vi "Actor Core.vi"(8 "error in":errorcluster, 11 "Actor in":refnum<class "EventLogger_Actor.lvclass">) -> (0 "error out":errorcluster, 3 "Actor out":refnum<class "Actor.lvclass">)   [LabVIEW 2014, in "EventLogger_Actor.lvlib" / "EventLogger_Actor.lvclass"]
uses:
  EventLogger_Actor.lvclass
  <vilib>/ActorFramework/Actor/Actor.lvclass
  EventLogger_Actor.lvclass/EventLogger_Actor.ctl
  <vilib>/ActorFramework/Actor/Actor.lvclass/Actor.ctl
  <vilib>/ActorFramework/Message Enqueuer/Message Enqueuer.lvclass/Message Enqueuer.ctl
  <vilib>/ActorFramework/Message Enqueuer/Init from Existing Queue.vi
  <vilib>/ActorFramework/Message Enqueuer/Enqueue.vi
  <vilib>/ActorFramework/Message Priority Queue/Priority Enqueue.vi
  <vilib>/ActorFramework/Message Enqueuer/Message Enqueuer.lvclass
  <vilib>/ActorFramework/Stop Msg/Stop Msg.lvclass
  EventLogger_Actor Messages/OpenLogs_Msg/OpenLogs_Msg.lvclass
panel:
  in  "ShowOnlyErrors":bool
  in  "Multicolumn Listbox":i32(listbox)
  out "StopLoop(Hidden)":bool
  in  "Stop":bool
  # "BSD 2-Clause License\n\nCopyright (c) 2018, Ajay www.digiajay.com\nAll rights reserved.\n\nRedistribution and use in source and binary forms, with or without\nmodification, are permitted provided that the following conditions are met:\n\n* Redistributions of source code must retain the above copyright notice, this\n  list of conditions and the following disclaimer.\n\n* Redistributions in binary form must reproduce the above copyright notice,\n  this list of conditions and the following disclaimer in the documentation\n  and/or other materials provided with the distribution.\n\nTHIS SOFTWARE IS PROVIDED BY THE COPYRIGHT HOLDERS AND CONTRIBUTORS \"AS IS\"\nAND ANY EXPRESS OR IMPLIED WARRANTIES, INCLUDING, BUT NOT LIMITED TO, THE\nIMPLIED WARRANTIES OF MERCHANTABILITY AND FITNESS FOR A PARTICULAR PURPOSE ARE\nDISCLAIMED. IN NO EVENT SHALL THE COPYRIGHT HOLDER OR CONTRIBUTORS BE LIABLE\nFOR ANY DIRECT, INDIRECT, INCIDENTAL, SPECIAL, EXEMPLARY, OR CONSEQUENTIAL\nDAMAGES (INCLUDING, BUT NOT LIMITED TO, PROCUREMENT OF SUBSTITUTE GOODS OR\nSERVICES; LOSS OF USE, DATA, OR PROFITS; OR BUSINESS INTERRUPTION) HOWEVER\nCAUSED AND ON ANY THEORY OF LIABILITY, WHETHER IN CONTRACT, STRICT LIABILITY,\nOR TORT (INCLUDING NEGLIGENCE OR OTHERWISE) ARISING IN ANY WAY OUT OF THE USE\nOF THIS SOFTWARE, EVEN IF ADVISED OF THE POSSIBILITY OF SUCH DAMAGE."
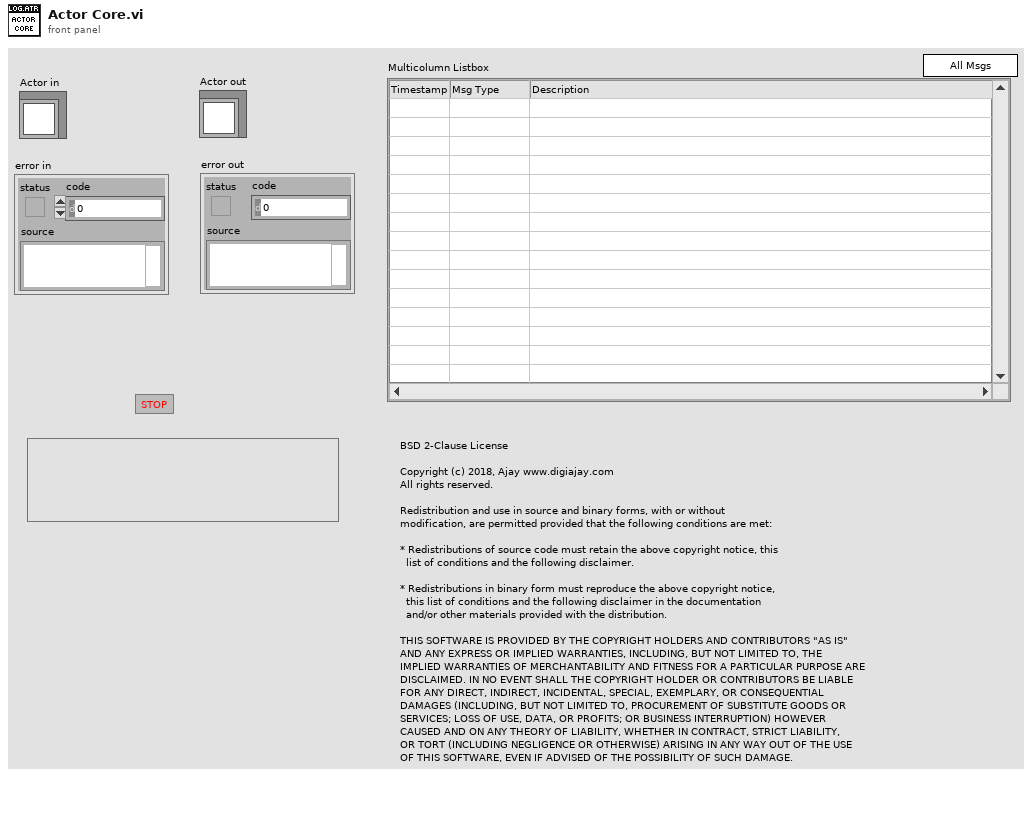
[diagram p1: front panel]
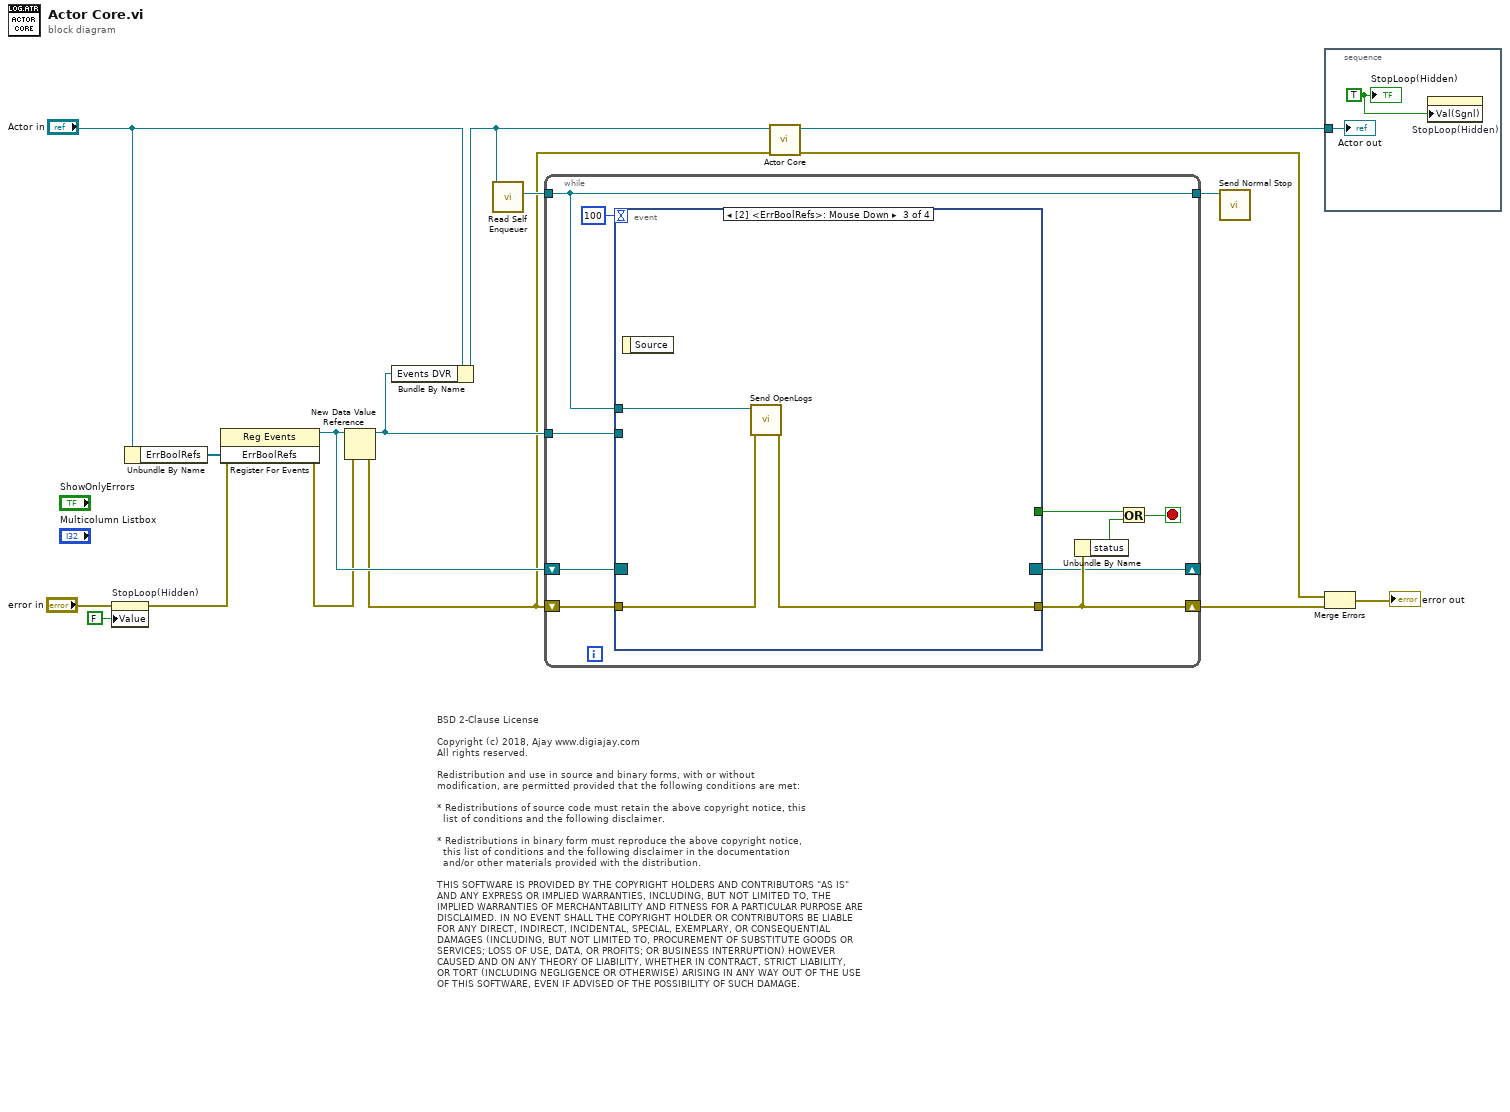
[diagram p0: block diagram]
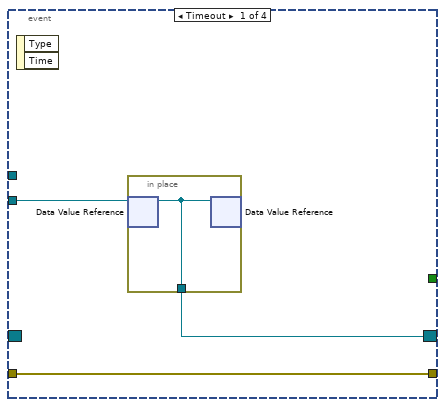
[diagram p2: hidden frame]
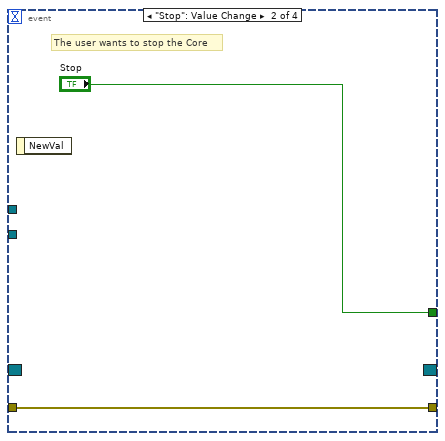
[diagram p3: hidden frame]
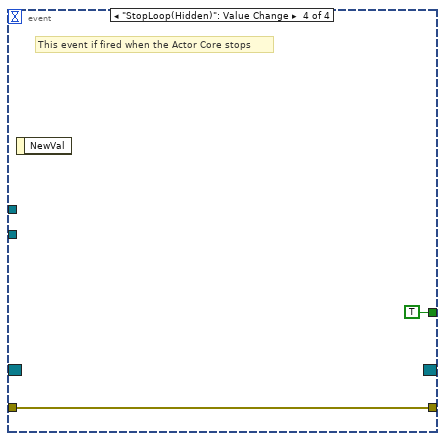
[diagram p4: hidden frame]
diagram:
  # "BSD 2-Clause License\n\nCopyright (c) 2018, Ajay www.digiajay.com\nAll rights reserved.\n\nRedistribution and use in source and binary forms, with or without\nmodification, are permitted provided that the following conditions are met:\n\n* Redistributions of source code must retain the above copyright notice, this\n  list of conditions and the following disclaimer.\n\n* Redistributions in binary form must reproduce the above copyright notice,\n  this list of conditions and the following disclaimer in the documentation\n  and/or other materials provided with the distribution.\n\nTHIS SOFTWARE IS PROVIDED BY THE COPYRIGHT HOLDERS AND CONTRIBUTORS \"AS IS\"\nAND ANY EXPRESS OR IMPLIED WARRANTIES, INCLUDING, BUT NOT LIMITED TO, THE\nIMPLIED WARRANTIES OF MERCHANTABILITY AND FITNESS FOR A PARTICULAR PURPOSE ARE\nDISCLAIMED. IN NO EVENT SHALL THE COPYRIGHT HOLDER OR CONTRIBUTORS BE LIABLE\nFOR ANY DIRECT, INDIRECT, INCIDENTAL, SPECIAL, EXEMPLARY, OR CONSEQUENTIAL\nDAMAGES (INCLUDING, BUT NOT LIMITED TO, PROCUREMENT OF SUBSTITUTE GOODS OR\nSERVICES; LOSS OF USE, DATA, OR PROFITS; OR BUSINESS INTERRUPTION) HOWEVER\nCAUSED AND ON ANY THEORY OF LIABILITY, WHETHER IN CONTRACT, STRICT LIABILITY,\nOR TORT (INCLUDING NEGLIGENCE OR OTHERWISE) ARISING IN ANY WAY OUT OF THE USE\nOF THIS SOFTWARE, EVEN IF ADVISED OF THE POSSIBILITY OF SUCH DAMAGE."
  n1 = property on="StopLoop(Hidden)" class="Bool (strict)"(error in="error in", "Value"=FALSE ("Stop")) -> ()  [unwired: 1 in, 2 out]
  n2 = Unbundle By Name("Actor in") -> ("ErrBoolRefs"=w4:refnum<vi>[])
  n3 = register-events(error in="error in", w4) -> (reference out=w7:refnum<event-registration>, error out=w1:errorcluster)  [unwired: 1 in]
  n4 = New Data Value Reference(data value=w7, error in=w1) -> (data value reference=w6:refnum<data-value>, error out=w3:errorcluster)
  n5 = Bundle By Name(cluster="Actor in", "Events DVR"=w6) -> (w8:refnum<class "EventLogger_Actor.lvclass">)
  n6 = call <vilib>:"Read Self Enqueuer.vi"("Actor"=w8) -> ("Self Enqueuer"=w10:refnum<class "Message Enqueuer.lvclass">)  [unwired: 10 in]
  n7 = while {
    tunnel: w10 -> [w16]
    shift-right: [w20] -> w15
    shift-left: w3 -> [w25]
    tunnel: [w16] -> w9
    shift-right: [w18] -> _
    shift-left: w7 -> [w19]
    tunnel: w6 -> [w17]
    stop <- w21 stop-if-true
    n8 = event shown="[2] <ErrBoolRefs>: Mouse Down" {
      selector: w19 -> [_ _ _ _]
      dyn-events: [w26 _ _ _] -> w18
      timeout: 100 -> [_ _ _ _]
      tunnel: w25 -> [w28 w31 w33 w35]
      tunnel: [w28 w31 w32 w35] -> w20
      tunnel: [_ "Stop" _ TRUE ("Stop")] -> w22
      tunnel: w17 -> [w27 _ _ _]
      tunnel: w16 -> [_ _ w34 _]
      event Timeout {
        n9 = event-data() -> ()  [unwired: 1 in, 2 out]
        n10 = in-place {
          in-place-border: [w29] -> w26
          n11 = in-place-dvr #1(w27) -> (w29:refnum<event-registration>)  [unwired: 1 out]
          n12 = in-place-dvr #1(w29) -> ()  [unwired: 2 out]
        }
      }
      event "Stop": Value Change {
        # "The user wants to stop the Core"
        n13 = event-data() -> ()  [unwired: 1 in, 1 out]
      }
      event Mouse Down {
        n14 = event-data() -> ()  [unwired: 1 in, 1 out]
        n15 = call "Send OpenLogs.vi"("error in (no error)"=w33, "Message Enqueuer"=w34) -> ("error out"=w32:errorcluster)  [unwired: 8 in, 1 out]
      }
      event "StopLoop(Hidden)": Value Change {
        # "This event if fired when the Actor Core stops"
        n16 = event-data() -> ()  [unwired: 1 in, 1 out]
      }
    }
    n17 = Unbundle By Name(w20) -> ("status"=w23:bool)
    n18 = Or(x=w22, y=w23) -> (x .or. y?=w21:bool)
  }
  n19 = call-parent "Actor Core.vi"("error in"=w3, "Actor in"=w8) -> ("error out"=w14:errorcluster, "Actor out"=w11:refnum<class "Actor.lvclass">)  [unwired: 8 in]
  n20 = call <vilib>:"Send Normal Stop.vi"("Message Enqueuer"=w9) -> ()  [unwired: 10 in, 1 out]
  n21 = stacked-sequence {
    tunnel: w11 -> [w38]
    frame #0 {
      w37 = TRUE ("StopLoop(Hidden)")
      n22 = property on="StopLoop(Hidden)" class="Bool (strict)"("Val(Sgnl)"=w37) -> ()  [unwired: 2 in, 2 out]
      "Actor out" <- w38
      "StopLoop(Hidden)" <- w37
    }
  }
  n23 = Merge Errors(w14, w15) -> (→"error out":errorcluster)
